vi "Test NES.vi"() -> ()   [LabVIEW 2019]
uses:
  <userlib>/LevyLab/Configuration/Configuration.lvclass
  src/Instrument.DAQ/Typedefs/PublicEvents--DAQ.getSweepWaveforms.ctl
  src/Instrument.DAQ/Instrument.DAQ.lvclass
  src/Instrument.DAQ/Typedefs/Results--Cluster.ctl
  src/Instrument.DAQ/Typedefs/PublicEvents--DAQ.getWaveforms.ctl
  src/Instrument.DAQ/Typedefs/Get State-enum.ctl
  src/Instrument.Lockin/Typedefs/Lockin.getAllData--Cluster.ctl
  src/Instrument.Lockin/Instrument.Lockin.lvclass
  src/Instrument UI.Lockin/Typedefs/UI.References.Graphs--Cluster.ctl
  src/Instrument UI.Lockin/Instrument UI.Lockin.lvclass
  src/Instrument UI.Lockin/Typedefs/UI.References.Clusters--Cluster.ctl
  src/Instrument UI.Lockin/Typedefs/UI.References.Booleans--Cluster.ctl
  src/Instrument UI.Lockin/Typedefs/UI.References--Cluster.ctl
  src/Generator/typedefs/Sweep.Pattern--Enum.ctl
  src/Generator/Generator.lvclass
  src/Generator/typedefs/Sweep.Channel--Cluster.ctl
  src/Generator/typedefs/Sweep.Channel--Cluster--Array.ctl
  src/Generator/typedefs/Sweep.Configuration--Cluster.ctl
  src/Instrument.DAQ/Typedefs/Configuration.LinkFrequencies--Cluster.ctl
  src/Instrument.DAQ/Typedefs/Configuration.DCLimit--Cluster.ctl
  src/Instrument.DAQ/Typedefs/Configuration.AmplitudeLimit--Cluster.ctl
  src/Instrument.DAQ/Typedefs/Channel.Gain--Cluster.ctl
  src/Instrument.DAQ/Typedefs/Channel.Gain--Cluster--Array.ctl
  src/Instrument.DAQ/Typedefs/Channel.GainsAndOffsets--Cluster.ctl
  src/Instrument.DAQ/Typedefs/Configuration.Prefilter--Cluster.ctl
  src/Instrument.DAQ/Typedefs/Simulation Mode--enum.ctl
  src/DAQmx/typedefs/DAQ.Calibration--Cluster.ctl
  src/DAQmx/DAQmx.lvclass
  src/DAQmx/typedefs/DAQ.Calibration--Cluster--Array.ctl
  src/Instrument.DAQ/Typedefs/DAQ.Config.Terminal Configuration--ring.ctl
  src/DAQmx/typedefs/DAQ.Config.AI.Coupling--enum.ctl
  src/DAQmx/typedefs/DAQ.Config.AI.Range--enum.ctl
  src/DAQmx/typedefs/DAQ.Config.AO.Range--enum.ctl
  src/Instrument.DAQ/Typedefs/DAQ.Configuration--Cluster.ctl
  src/Instrument.DAQ/Typedefs/DAQ.Configuration--Cluster--Array.ctl
  src/Instrument.DAQ/Typedefs/REF.Channel--Cluster.ctl
  src/Instrument.DAQ/Typedefs/REF.Channel--Cluster--Array.ctl
  src/Instrument.DAQ/Typedefs/AI.Channel--Cluster.ctl
  src/Instrument.DAQ/Typedefs/AI.Channel--Cluster--Array.ctl
  src/Generator/typedefs/AO.Channel.Function--Enum.ctl
  src/Generator/typedefs/AO.Channel--Cluster.ctl
  src/Generator/typedefs/AO.Channel--Cluster--Array.ctl
  src/Instrument.DAQ/Typedefs/Configuration.Channels--Cluster.ctl
  src/Instrument UI.Lockin/Typedefs/UI.Configuration--Cluster.ctl
  <vilib>/measure/NI_MABase.lvlib
  <userlib>/LevyLab/Lockin-Multichannel/Instrument.DAQ/Typedefs/-DAQ.Sampling.Fs Mode--enum.ctl
  <userlib>/LevyLab/Lockin-Multichannel/Instrument.DAQ/Typedefs/-DAQ.Sampling.Sampling--Cluster.ctl
  <userlib>/LevyLab/Lockin-Multichannel/Instrument.DAQ/Typedefs/-DAQ.Sampling--Cluster.ctl
panel:
  out "i":i32
  out "Total Time (BBN, In Place, In Place Bundle) (s)":dbl[](array[numeric]) format="%#_6p"
  out "Average Time (BBN, In Place, In Place Bundle) (s)":dbl[](array[numeric]) format="%#_6p"
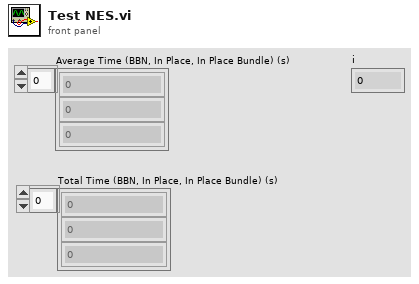
[diagram p1: front panel]
types:
  T1 = typedef "Instrument.Lockin.lvlib/Instrument.DAQ.lvclass/Get State-enum.ctl" = enum16{"idle", "created", "started", "stopped", "sweeping"}
  T2 = typedef "Instrument.Lockin.lvlib/Instrument UI.Lockin.lvclass/UI.Configuration--Cluster.ctl" = cluster{"Channels":T3, "DAQ":cluster{"Configuration":T11, "cfg.Sampling":T17, "Calibration":T20, "Simulation mode":T22}, "PreFilter":T23, "Amplifers":T24, "Limit Amplitude":T27, "Limit DC":T28, "Link Frequencies":T29, "Aux Channel":tag, "Sweep":T30, "Plot":cluster{"visibility.AI":bool[], "visibility.AO":bool[], "visibility.Lockin":bool[]}}
  T3 = typedef "Instrument.Lockin.lvlib/Instrument.DAQ.lvclass/Configuration.Channels--Cluster.ctl" = cluster{"Cfg_AO":T4, "Cfg_AI":T7, "Cfg_REF":T9}
  T4 = typedef "Generator.lvclass/AO.Channel--Cluster--Array.ctl" = T5[]
  T5 = typedef "Generator.lvclass/AO.Channel--Cluster.ctl" = cluster{"Enable?":bool, "Channel":i32, "Amplitude":dbl, "Offset":dbl, "Frequency":dbl, "Phase":dbl, "Function":T6, "Sweeping?":bool, "Limit AC":bool, "Limit DC?":bool}
  T6 = typedef "Generator.lvclass/AO.Channel.Function--Enum.ctl" = enum16{"Sine", "Triangle", "Square"}
  T7 = typedef "Instrument.Lockin.lvlib/Instrument.DAQ.lvclass/AI.Channel--Cluster--Array.ctl" = T8[]
  T8 = typedef "Instrument.Lockin.lvlib/Instrument.DAQ.lvclass/AI.Channel--Cluster.ctl" = cluster{"Enable?":bool, "Channel":i32, "References":i32[]}
  T9 = typedef "Instrument.Lockin.lvlib/Instrument.DAQ.lvclass/REF.Channel--Cluster--Array.ctl" = T10[]
  T10 = typedef "Instrument.Lockin.lvlib/Instrument.DAQ.lvclass/REF.Channel--Cluster.ctl" = cluster{"Enable?":bool, "Channel":i32, "Frequency":dbl, "Phase":dbl, "TC":dbl, "Roll-Off":i32}
  T11 = typedef "Instrument.Lockin.lvlib/Instrument.DAQ.lvclass/DAQ.Configuration--Cluster--Array.ctl" = T12[]
  T12 = typedef "Instrument.Lockin.lvlib/Instrument.DAQ.lvclass/DAQ.Configuration--Cluster.ctl" = cluster{"Device":string, "AO.Ch":string, "AO.Range":T13, "AI.Ch":string, "AI.Range":T14, "AI.Coupling":T15, "AI terminal config":T16, "AO terminal config":T16}
  T13 = typedef "DAQmx.lvclass/DAQ.Config.AO.Range--enum.ctl" = enum16{"±0.1", "±1.0", "±10.0", ""}
  T14 = typedef "DAQmx.lvclass/DAQ.Config.AI.Range--enum.ctl" = enum16{"±0.316", "±1.00", "±3.16", "±10.0", "±31.6", "±42.4", ""}
  T15 = typedef "DAQmx.lvclass/DAQ.Config.AI.Coupling--enum.ctl" = u16
  T16 = typedef "DAQmx.lvclass/DAQ.Config.Terminal Configuration--ring.ctl" = i32
  T17 = typedef "Instrument.Lockin.lvlib/Instrument.DAQ.lvclass/-DAQ.Sampling--Cluster.ctl" = cluster{"Sampling":T18, "sample mode":i32, "Fs Mode":T19, "Fs Multiplier":dbl, "Refresh Rate (Hz)":dbl, "Decimation.PreDSP":i32, "Decimation.PostDSP":i32, "Fs.Output":dbl}
  T18 = typedef "Instrument.Lockin.lvlib/Instrument.DAQ.lvclass/-DAQ.Sampling.Sampling--Cluster.ctl" = cluster{"Fs":dbl, "#s":i32}
  T19 = typedef "Instrument.Lockin.lvlib/Instrument.DAQ.lvclass/-DAQ.Sampling.Fs Mode--enum.ctl" = enum16{"Manual", "Auto Fs", "Max Fs"}
  T20 = typedef "DAQmx.lvclass/DAQ.Calibration--Cluster--Array.ctl" = T21[]
  T21 = typedef "DAQmx.lvclass/DAQ.Calibration--Cluster.ctl" = cluster{"Active Device":string, "SelfCal.LastDate/Time":dbl, "SelfCal.LastTemp":dbl, "DevTemp":dbl, "calibration due?":bool}
  T22 = typedef "Instrument.Lockin.lvlib/Instrument.DAQ.lvclass/Simulation Mode--enum.ctl" = enum16{"AI = HW simulated", "AI = noise*AO", "AI = waveguide"}
  T23 = typedef "Instrument.Lockin.lvlib/Instrument.DAQ.lvclass/Configuration.Prefilter--Cluster.ctl" = cluster{"60 Hz":bool, "Low Pass":bool, "Low Pass Cutoff (Hz)":dbl}
  T24 = typedef "Instrument.Lockin.lvlib/Instrument.DAQ.lvclass/Channel.GainsAndOffsets--Cluster.ctl" = cluster{"Offset_AI":T25, "Gain_AI":T25, "Gain_AO":T25}
  T25 = typedef "Instrument.Lockin.lvlib/Instrument.DAQ.lvclass/Channel.Gain--Cluster--Array.ctl" = T26[]
  T26 = typedef "Instrument.Lockin.lvlib/Instrument.DAQ.lvclass/Channel.Gain--Cluster.ctl" = cluster{"Channel":string, "Gain":dbl}
  T27 = typedef "Instrument.Lockin.lvlib/Instrument.DAQ.lvclass/Configuration.AmplitudeLimit--Cluster.ctl" = cluster{"Limit?":bool, "Limit (V)":dbl}
  T28 = typedef "Instrument.Lockin.lvlib/Instrument.DAQ.lvclass/Configuration.DCLimit--Cluster.ctl" = cluster{"Limit?":bool, "Limit (V)":dbl}
  T29 = typedef "Instrument.Lockin.lvlib/Instrument.DAQ.lvclass/Configuration.LinkFrequencies--Cluster.ctl" = cluster{"Link?":bool, "Frequency (Hz)":dbl}
  T30 = typedef "Generator.lvclass/Sweep.Configuration--Cluster.ctl" = cluster{"Sweep Time (s)":dbl, "Initial Wait (s)":dbl, "Return to Start":bool, "Channels":T31}
  T31 = typedef "Generator.lvclass/Sweep.Channel--Cluster--Array.ctl" = T32[]
  T32 = typedef "Generator.lvclass/Sweep.Channel--Cluster.ctl" = cluster{"Enable?":bool, "Channel":u16, "Start":dbl, "End":dbl, "Pattern":T33, "Table":dbl[]}
  T33 = typedef "Generator.lvclass/Sweep.Pattern--Enum.ctl" = enum16{"Ramp /", "Ramp /\\", "Smooth Ramp _/", "Smooth Ramp _/\\_", "Table"}
  T34 = typedef "Instrument.Lockin.lvlib/Instrument UI.Lockin.lvclass/UI.References--Cluster.ctl" = cluster{"Booleans":T35, "Clusters":T36, "Graphs":T37}
  T35 = typedef "Instrument.Lockin.lvlib/Instrument UI.Lockin.lvclass/UI.References.Booleans--Cluster.ctl" = cluster{"Start":refnum<vi>, "Pause":refnum<vi>, "Reset":refnum<vi>, "Trigger":refnum<vi>, "Help":refnum<vi>, "Close":refnum<vi>, "Start Sweep":refnum<vi>, "Stop Sweep":refnum<vi>}
  T36 = typedef "Instrument.Lockin.lvlib/Instrument UI.Lockin.lvclass/UI.References.Clusters--Cluster.ctl" = cluster{"AO Channels":refnum<vi>, "AI Channels":refnum<vi>, "REF Channels":refnum<vi>, "DAQ Config":refnum<vi>, "Sweep Channels":refnum<vi>, "Cal Info":refnum<vi>}
  T37 = typedef "Instrument.Lockin.lvlib/Instrument UI.Lockin.lvclass/UI.References.Graphs--Cluster.ctl" = cluster{"AI Graph":refnum<vi>, "AO Graph":refnum<vi>, "Lockin 1":refnum<vi>, "Lockin 2":refnum<vi>, "XY Graph":refnum<vi>, "Sweep X Graph":refnum<vi>, "Sweep Y Graph":refnum<vi>, "Sweep AI Graph":refnum<vi>, "Sweep AO Graph":refnum<vi>, "PS WFGraph":refnum<vi>, "PS Chart":refnum<vi>}
  T38 = typedef "Instrument.Lockin.lvlib/Instrument.Lockin.lvclass/Lockin.getAllData--Cluster.ctl" = cluster{"DAQ State":T1, "Waveforms":T39, "Results":T40, "SweepWaveforms":T41}
  T39 = typedef "Instrument.Lockin.lvlib/Instrument.DAQ.lvclass/PublicEvents--DAQ.getWaveforms.ctl" = cluster{"AO_wfm":waveform(dbl)[], "AI_wfm":waveform(dbl)[], "Ref_X_wfm":waveform(dbl)[], "Ref_Y_wfm":waveform(dbl)[], "X_wfm":waveform(dbl)[], "Y_wfm":waveform(dbl)[]}
  T40 = typedef "Instrument.Lockin.lvlib/Instrument.DAQ.lvclass/Results--Cluster.ctl" = cluster{"Time Stamp":timestamp, "Results (Dictionary)":cluster{"key":string, "value":dbl}[]}
  T41 = typedef "Instrument.Lockin.lvlib/Instrument.DAQ.lvclass/PublicEvents--DAQ.getSweepWaveforms.ctl" = cluster{"AO_wfm":waveform(dbl)[], "AI_wfm":waveform(dbl)[], "X_wfm":waveform(dbl)[], "Y_wfm":waveform(dbl)[]}
  T42 = cluster{"i":i32, "Configuration":refnum<class "Configuration.lvclass">, "UI Config":T2, "DAQ state":T1, "getAll":T38, "References":T34, "Message":cluster{"Command":variant, "Data":variant}, "Plot Names":string[], "Front Panel":refnum<vi>, "update graphs":bool}
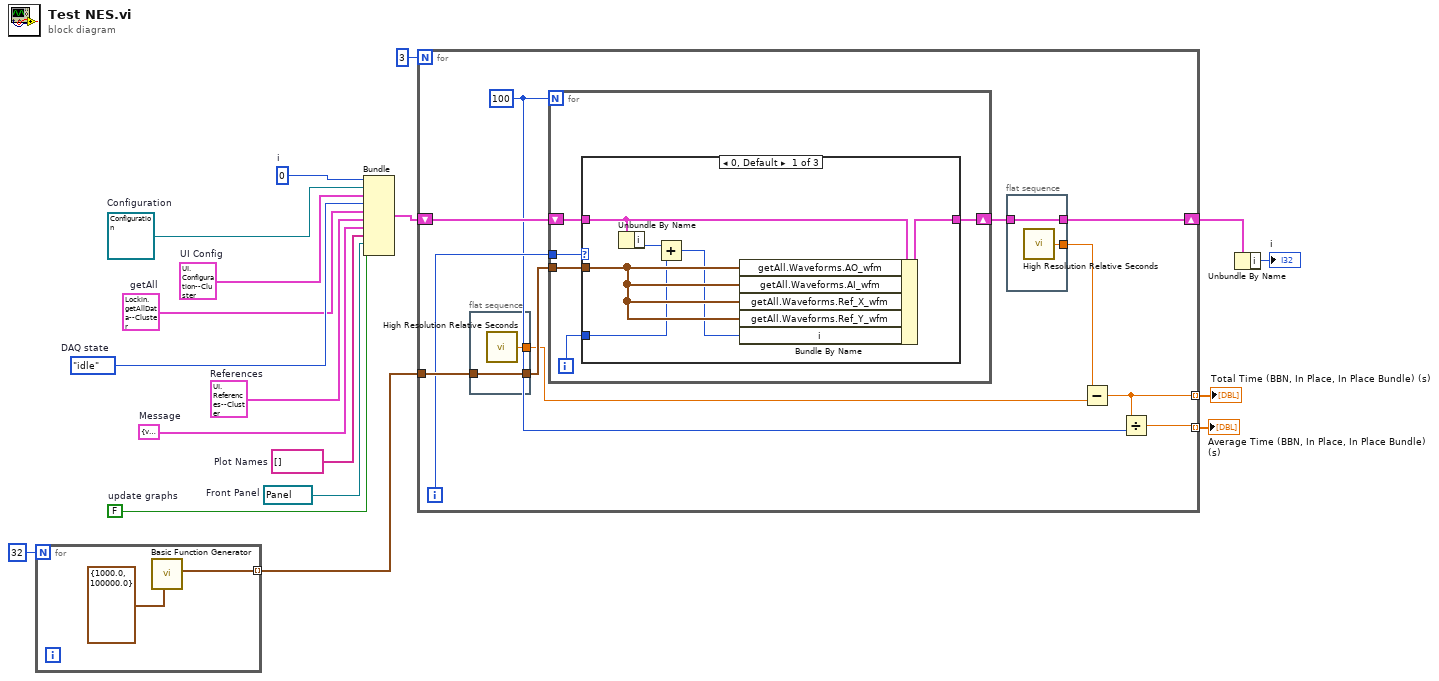
[diagram p0: block diagram]
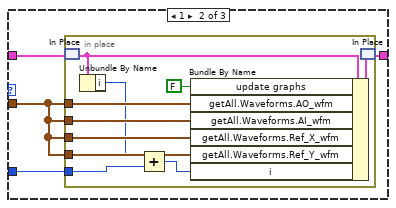
[diagram p2: hidden frame]
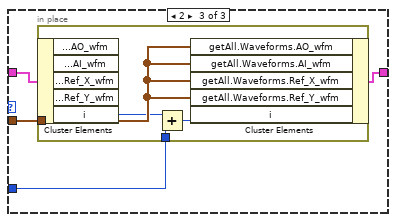
[diagram p3: hidden frame]
diagram:
  w3 = 0  # i
  w10 = FALSE  # update graphs
  w12 = Get_State-enum."idle"  # DAQ state
  w13 = refnum<vi> refnum  # Front Panel
  w15 = T2 {"Channels"={"Cfg_AO"=[], "Cfg_AI"=[], "Cfg_REF"=[]}, "DAQ"={"Configuration"=[], "cfg.Sampling"={"Sampling"={"Fs"=0.0, "#s"=0}, "sample mode"=0, "Fs Mode"=enum."Manual", "Fs Multiplier"=0.0, "Refresh Rate (Hz)"=0.0, "Decimation.PreDSP"=0, "Decimation.PostDSP"=0, "Fs.Output"=204789.0}, "Calibration"=[], "Simulation mode"=enum."AI = HW simulated"}, "PreFilter"={"60 Hz"=FALSE, "Low Pass"=FALSE, "Low Pass Cutoff (Hz)"=0.0}, "Amplifers"={"Offset_AI"=[], "Gain_AI"=[], "Gain_AO"=[]}, "Limit Amplitude"={"Limit?"=FALSE, "Limit (V)"=0.0}, "Limit DC"={"Limit?"=FALSE, "Limit (V)"=0.0}, "Link Frequencies"={"Link?"=FALSE, "Frequency (Hz)"=0.0}, "Aux Channel"="", "Sweep"={"Sweep Time (s)"=0.0, "Initial Wait (s)"=0.0, "Return to Start"=FALSE, "Channels"=[]}, "Plot"={"visibility.AI"=[], "visibility.AO"=[], "visibility.Lockin"=[]}}  # UI Config
  w14 = string[] []  # Plot Names
  w18 = T34 {"Booleans"={"Start"=refnum, "Pause"=refnum, "Reset"=refnum, "Trigger"=refnum, "Help"=refnum, "Close"=refnum, "Start Sweep"=refnum, "Stop Sweep"=refnum}, "Clusters"={"AO Channels"=refnum, "AI Channels"=refnum, "REF Channels"=refnum, "DAQ Config"=refnum, "Sweep Channels"=refnum, "Cal Info"=refnum}, "Graphs"={"AI Graph"=refnum, "AO Graph"=refnum, "Lockin 1"=refnum, "Lockin 2"=refnum, "XY Graph"=refnum, "Sweep X Graph"=refnum, "Sweep Y Graph"=refnum, "Sweep AI Graph"=refnum, "Sweep AO Graph"=refnum, "PS WFGraph"=refnum, "PS Chart"=refnum}}  # References
  w16 = cluster{"Command":variant, "Data":variant} {"Command"=variant, "Data"=variant}  # Message
  w11 = T38 {"DAQ State"=enum."idle", "Waveforms"={"AO_wfm"=[], "AI_wfm"=[], "Ref_X_wfm"=[], "Ref_Y_wfm"=[], "X_wfm"=[], "Y_wfm"=[]}, "Results"={"Time Stamp"=timestamp(0 s since 1904-01-01), "Results (Dictionary)"=[]}, "SweepWaveforms"={"AO_wfm"=[], "AI_wfm"=[], "X_wfm"=[], "Y_wfm"=[]}}  # getAll
  w17 = refnum<class "Configuration.lvclass"> refnum  # Configuration
  n1 = for {
    N: 32 -> [_]
    tunnel: [w19] -> w7 mode=indexing
    n2 = call <vilib>:"Basic Function Generator.vi"("sampling info"=cluster{"Fs":dbl, "#s":dbl} {"Fs"=1000.0, "#s"=100000.0}) -> ("signal out"=w19:waveform(dbl))  [unwired: 8 in, 2 out]
  }
  n3 = Bundle("i"=w3, "Configuration"=w17, "UI Config"=w15, "DAQ state"=w12, "getAll"=w11, "References"=w18, "Message"=w16, "Plot Names"=w14, "Front Panel"=w13, "update graphs"=w10) -> (w9:T42)  [unwired: 1 in]
  n4 = for {
    N: 3 -> [_]
    tunnel: w7 -> [w29]
    shift-right: [w27] -> w2
    shift-left: w9 -> [w31]
    tunnel: [w23] -> w5 mode=indexing
    tunnel: [w21] -> w4 mode=indexing
    i -> [w26]
    w22 = 100
    n5 = flat-sequence {
      tunnel: w29 -> [w35]
      tunnel: [w35] -> w30
      tunnel: [w34] -> w24
      frame #0 {
        n6 = call <vilib>:"High Resolution Relative Seconds.vi"() -> ("relative seconds"=w34:dbl)
      }
    }
    n7 = for {
      N: w22 -> [_]
      tunnel: w30 -> [w39]
      shift-right: [w38] -> w28
      shift-left: w31 -> [w40]
      tunnel: w26 -> [w37]
      i -> [w36]
      n8 = case shown="0, Default" w37 {
        tunnel: w40 -> [w44 w50 w64]
        tunnel: w39 -> [w45 w49 w62]
        tunnel: [w46 w48 w63] -> w38
        tunnel: w36 -> [w41 w47 w61]
        frame 0, Default {
          n9 = Unbundle By Name(w44) -> ("i"=w43:i32)
          n10 = Add(x=w43, y=w41) -> (x+y=w42:i32)
          n11 = Bundle By Name(cluster=w44, "getAll.Waveforms.AO_wfm"=w45, "getAll.Waveforms.AI_wfm"=w45, "getAll.Waveforms.Ref_X_wfm"=w45, "getAll.Waveforms.Ref_Y_wfm"=w45, "i"=w42) -> (w46:T42)
        }
        frame 1 {
          n12 = in-place {
            in-place-border: w49 -> [w60]
            in-place-border: w49 -> [w59]
            in-place-border: w49 -> [w58]
            in-place-border: w49 -> [w57]
            in-place-border: w47 -> [w51]
            n13 = in-place-match #1(w50) -> (w54:T42)
            n14 = Unbundle By Name(w54) -> ("i"=w53:i32)
            n15 = Add(x=w53, y=w51) -> (x+y=w52:i32)
            n16 = Bundle By Name(cluster=w54, "update graphs"=FALSE, "getAll.Waveforms.AO_wfm"=w57, "getAll.Waveforms.AI_wfm"=w60, "getAll.Waveforms.Ref_X_wfm"=w59, "getAll.Waveforms.Ref_Y_wfm"=w58, "i"=w52) -> (w55:T42)
            n17 = in-place-match #1(w55) -> (w48:T42)
          }
        }
        frame 2 {
          n18 = in-place {
            in-place-border: w62 -> [w68]
            in-place-border: w61 -> [w66]
            n19 = in-place-cluster #2(w64) -> ("i"=w67:i32)  [unwired: 4 out]
            n20 = Add(x=w67, y=w66) -> (x+y=w65:i32)
            n21 = in-place-cluster #2("getAll.Waveforms.AO_wfm"=w68, "getAll.Waveforms.AI_wfm"=w68, "getAll.Waveforms.Ref_X_wfm"=w68, "getAll.Waveforms.Ref_Y_wfm"=w68, "i"=w65) -> (w63:T42)
          }
        }
      }
    }
    n22 = flat-sequence {
      tunnel: w28 -> [w33]
      tunnel: [w33] -> w27
      tunnel: [w32] -> w25
      frame #0 {
        n23 = call <vilib>:"High Resolution Relative Seconds.vi"() -> ("relative seconds"=w32:dbl)
      }
    }
    n24 = Subtract(x=w25, y=w24) -> (x-y=w21:dbl)
    n25 = Divide(x=w21, y=w22) -> (x/y=w23:dbl)
  }
  "Average Time (BBN, In Place, In Place Bundle) (s)" <- w5
  "Total Time (BBN, In Place, In Place Bundle) (s)" <- w4
  n26 = Unbundle By Name(w2) -> ("i"=→"i":i32)
